vi "7.0-Main Non GUI.vi"(1 "Begin (for Flow)":bool) -> (0 "End Program":bool)   [LabVIEW 2010]
uses:
  7.0-OCU State.ctl
  7.0-Global.vi
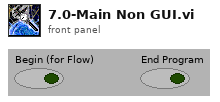
[diagram p1: front panel]
types:
  T1 = typedef "7.0-OCU State.ctl" = enum16{"Startup", "Self Test", "Manual Mode", "Auto Mode", "Plan Mission", "Shutdown"}
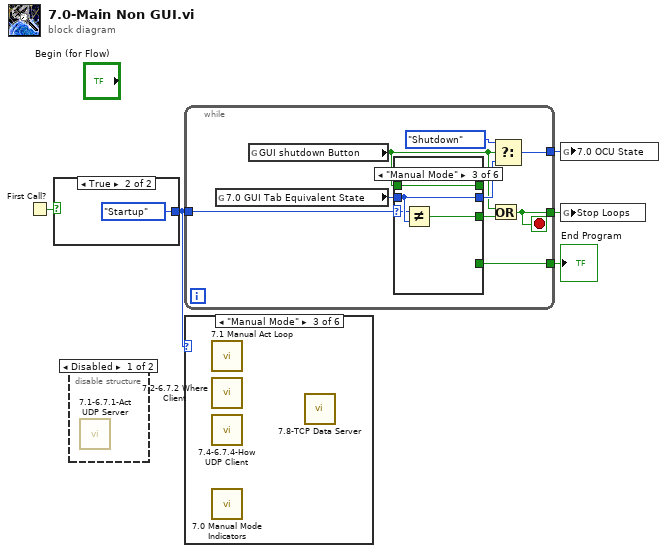
[diagram p0: block diagram]
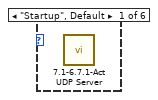
[diagram p3: hidden frame]
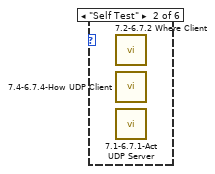
[diagram p4: hidden frame]
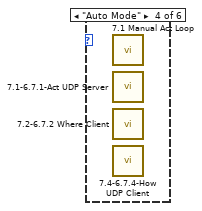
[diagram p5: hidden frame]
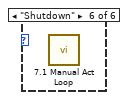
[diagram p7: hidden frame]
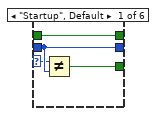
[diagram p8: hidden frame]
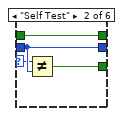
[diagram p9: hidden frame]
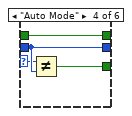
[diagram p10: hidden frame]
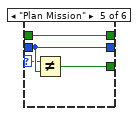
[diagram p11: hidden frame]
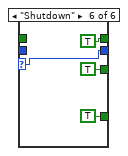
[diagram p12: hidden frame]
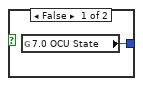
[diagram p13: hidden frame]
diagram:
  n1 = First Call?() -> (First Call?: T/F=w5:bool)
  n2 = case shown="True" w5 {
    tunnel: [w6 7.0-OCU_State."Startup" ("7.0 OCU State")] -> w2
    frame False {
      n3 = global read "7.0-Global.vi" "7.0 OCU State"() -> (w6:T1)
    }
    frame True {
    }
  }
  n4 = disable-structure shown="Disabled" {
    frame Disabled {
      n5 = call "7.1-6.7.1-Act UDP Server.vi"() -> ()  [unwired: 12 in]
    }
    frame Enabled {
    }
  }
  n6 = while {
    tunnel: w2 -> [w16]
    tunnel: [w14] -> w4
    tunnel: [w12] -> w3
    tunnel: [w8] -> w1
    stop <- w8 stop-if-true
    n7 = global read "7.0-Global.vi" "7.0 GUI Tab Equivalent State"() -> (w15:T1)
    n8 = global read "7.0-Global.vi" "GUI shutdown Button"() -> (w9:bool)
    n9 = case shown="\"Manual Mode\"" w16 {
      selector: w16 -> [w18 w22 w26 w30 w34 w38]
      tunnel: [_ _ _ _ _ TRUE] -> w14
      tunnel: [w20 w24 w28 w32 w36 TRUE] -> _
      tunnel: w9 -> [w20 w24 w28 w32 w36 _]
      tunnel: w15 -> [w19 w23 w27 w31 w35 _]
      tunnel: [w19 w23 w27 w31 w35 w38] -> w13
      tunnel: [w17 w21 w25 w29 w33 TRUE] -> w10
      frame "Startup", Default {
        n10 = Not Equal?(x=w18, y=w19) -> (x != y?=w17:bool)
      }
      frame "Self Test" {
        n11 = Not Equal?(x=w22, y=w23) -> (x != y?=w21:bool)
      }
      frame "Manual Mode" {
        n12 = Not Equal?(x=w26, y=w27) -> (x != y?=w25:bool)
      }
      frame "Auto Mode" {
        n13 = Not Equal?(x=w30, y=w31) -> (x != y?=w29:bool)
      }
      frame "Plan Mission" {
        n14 = Not Equal?(x=w34, y=w35) -> (x != y?=w33:bool)
      }
      frame "Shutdown" {
      }
    }
    n15 = Or(x=w9, y=w10) -> (x .or. y?=w8:bool)
    n16 = Select(t=7.0-OCU_State."Shutdown", s=w9, f=w13) -> (s? t:f=w12:T1)
  }
  "End Program" <- w4
  n17 = case shown="\"Manual Mode\"" w2 {
    frame "Startup", Default {
      n18 = call "7.1-6.7.1-Act UDP Server.vi"() -> ()  [unwired: 12 in]
    }
    frame "Self Test" {
      n19 = call "7.2-6.7.2 Where Client.vi"() -> ()  [unwired: 7 in]
      n20 = call "7.4-6.7.4-How UDP Client.vi"() -> ()  [unwired: 7 in]
      n21 = call "7.1-6.7.1-Act UDP Server.vi"() -> ()  [unwired: 12 in]
    }
    frame "Manual Mode" {
      n22 = call "7.1 Manual Act Loop.vi"() -> ()  [unwired: 12 in]
      n23 = call "7.2-6.7.2 Where Client.vi"() -> ()  [unwired: 7 in]
      n24 = call "7.4-6.7.4-How UDP Client.vi"() -> ()  [unwired: 7 in]
      n25 = call "7.0 Manual Mode Indicators.vi"() -> ()  [unwired: 12 in]
      n26 = call "7.8-TCP Data Server.vi"() -> ()  [unwired: 12 in]
    }
    frame "Auto Mode" {
      n27 = call "7.1 Manual Act Loop.vi"() -> ()  [unwired: 12 in]
      n28 = call "7.1-6.7.1-Act UDP Server.vi"() -> ()  [unwired: 12 in]
      n29 = call "7.2-6.7.2 Where Client.vi"() -> ()  [unwired: 7 in]
      n30 = call "7.4-6.7.4-How UDP Client.vi"() -> ()  [unwired: 7 in]
    }
    frame "Plan Mission" {
    }
    frame "Shutdown" {
      n31 = call "7.1 Manual Act Loop.vi"() -> ()  [unwired: 12 in]
    }
  }
  n32 = global write "7.0-Global.vi" "7.0 OCU State"(w3) -> ()
  n33 = global write "7.0-Global.vi" "Stop Loops"(w1) -> ()
